vi "Eth Status Manager Init.vi"(8 "error in (no error)":errorcluster, 11 "Data Buffer Length":i32=1000) -> (0 "error out":errorcluster, 3 "Status Reference":T1)   [LabVIEW 2019, in "Eth Status.lvlib"]
uses:
  Eth Status.lvlib
  Ctl/Status.ctl
  MB_TCP2/MB_TCP_State.ctl
  MB_TCP2/MB_TCP.lvclass
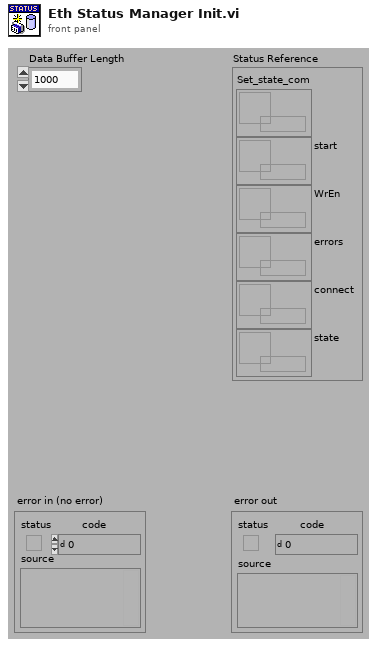
[diagram p1: front panel]
types:
  T1 = typedef "Eth Status.lvlib/Status.ctl" = cluster{"Set_state_com":refnum<data-value>, "start":refnum<data-value>, "WrEn":refnum<data-value>, "errors":refnum<data-value>, "connect":refnum<data-value>, "state":refnum<data-value>}
  T2 = typedef "MB_TCP.lvclass/MB_TCP_State.ctl" = enum8{"initialization", "redefine", "standby", "connect", "wait to reconnect", "wait to reset timeout", "configure", "requests", "close connection", "stop"}
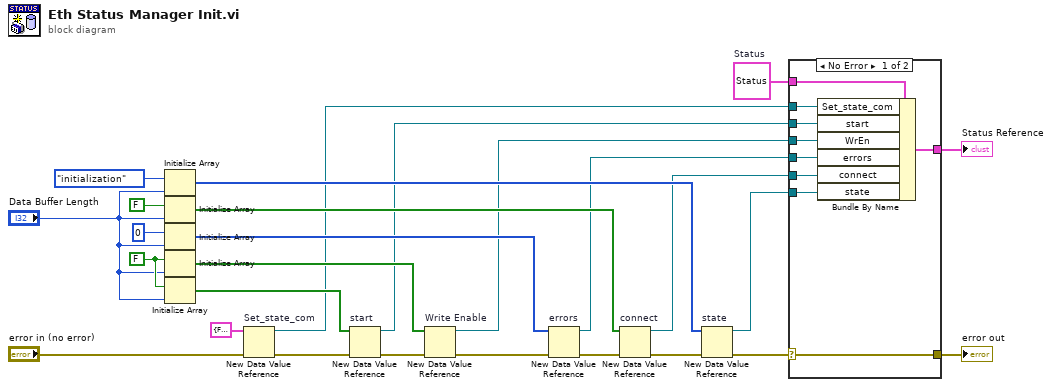
[diagram p0: block diagram]
diagram:
  w19 = FALSE
  w27 = T1 {"Set_state_com"=refnum, "start"=refnum, "WrEn"=refnum, "errors"=refnum, "connect"=refnum, "state"=refnum}  # Status
  n1 = Initialize Array(MB_TCP_State."initialization" ("MB_TCP_State"), "Data Buffer Length") -> (w13:T2[])
  n2 = Initialize Array(FALSE, "Data Buffer Length") -> (w18:bool[])
  n3 = Initialize Array(0, "Data Buffer Length") -> (w26:i32[])
  n4 = Initialize Array(w19, "Data Buffer Length") -> (w20:bool[])
  n5 = Initialize Array(w19, "Data Buffer Length") -> (w24:bool[])
  n6 = New Data Value Reference "Set_state_com"(data value=cluster{"Start":bool, "WrEn":bool, "Stop":bool} {"Start"=FALSE, "WrEn"=FALSE, "Stop"=FALSE} ("Set_state_com"), error in="error in (no error)") -> (data value reference=w1:refnum<data-value>, error out=w4:errorcluster)
  n7 = New Data Value Reference "start"(data value=w24, error in=w4) -> (data value reference=w11:refnum<data-value>, error out=w17:errorcluster)
  n8 = New Data Value Reference "Write Enable"(data value=w20, error in=w17) -> (data value reference=w10:refnum<data-value>, error out=w3:errorcluster)
  n9 = New Data Value Reference "errors"(data value=w26, error in=w3) -> (data value reference=w9:refnum<data-value>, error out=w12:errorcluster)
  n10 = New Data Value Reference "connect"(data value=w18, error in=w12) -> (data value reference=w8:refnum<data-value>, error out=w7:errorcluster)
  n11 = New Data Value Reference "state"(data value=w13, error in=w7) -> (data value reference=w6:refnum<data-value>, error out=w23:errorcluster)
  n12 = case shown="No Error" w23 {
    selector: w23 -> [w35 w37]
    tunnel: w27 -> [w29 w38]
    tunnel: [w36 w38] -> w25
    tunnel: [w35 w37] -> w22
    tunnel: w11 -> [w34 _]
    tunnel: w10 -> [w33 _]
    tunnel: w9 -> [w32 _]
    tunnel: w8 -> [w31 _]
    tunnel: w6 -> [w30 _]
    tunnel: w1 -> [w28 _]
    frame No Error {
      n13 = Bundle By Name(cluster=w29, "Set_state_com"=w28, "start"=w34, "WrEn"=w33, "errors"=w32, "connect"=w31, "state"=w30) -> (w36:T1)
    }
    frame Error {
    }
  }
  "error out" <- w22
  "Status Reference" <- w25
